vi "asc转换.vi"(11 "输入数据":u16) -> (0 "数值位 5":u8 format="%x", 1 "数值位 4":u8 format="%x", 2 "数值位 3":u8 format="%x", 3 "数值位 2":u8 format="%x")   [LabVIEW 2016]
panel:
  in  "数值 1":u8 format="%x"
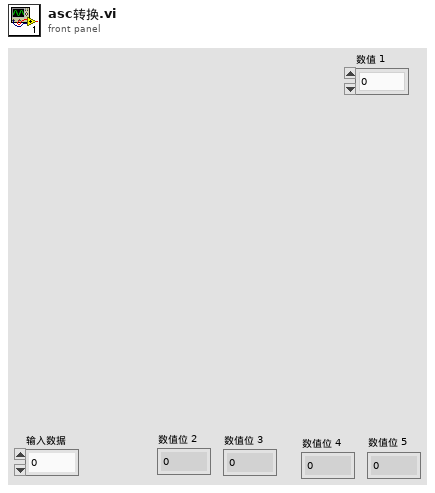
[diagram p1: front panel]
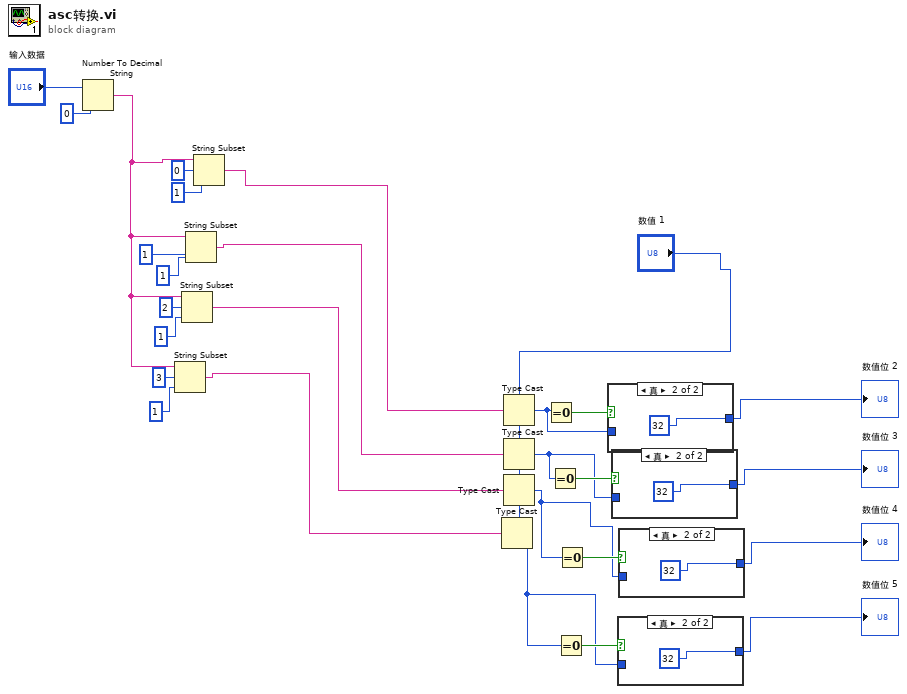
[diagram p0: block diagram]
diagram:
  n1 = Number To Decimal String(number="输入数据", width (-)=i16 0 ("宽度(-)")) -> (decimal integer string=w20:string)
  n2 = String Subset(string=w20, offset (0)=3 ("偏移量(0)"), length (rest)=1 ("长度（剩余）")) -> (substring=w14:string)
  n3 = String Subset(string=w20, offset (0)=2 ("偏移量(0)"), length (rest)=1 ("长度（剩余）")) -> (substring=w15:string)
  n4 = String Subset(string=w20, offset (0)=1 ("偏移量(0)"), length (rest)=1 ("长度（剩余）")) -> (substring=w16:string)
  n5 = String Subset(string=w20, offset (0)=0 ("偏移量(0)"), length (rest)=1 ("长度（剩余）")) -> (substring=w24:string)
  n6 = Type Cast(type="数值 1", x=w14) -> (*(type *) &x=w5:u8)
  n7 = Type Cast(type="数值 1", x=w24) -> (*(type *) &x=w11:u8)
  n8 = Type Cast(type="数值 1", x=w16) -> (*(type *) &x=w7:u8)
  n9 = Type Cast(type="数值 1", x=w15) -> (*(type *) &x=w6:u8)
  n10 = Equal To 0?(x=w11) -> (x = 0?=w13:bool)
  n11 = Equal To 0?(x=w7) -> (x = 0?=w10:bool)
  n12 = Equal To 0?(x=w5) -> (x = 0?=w8:bool)
  n13 = Equal To 0?(x=w6) -> (x = 0?=w9:bool)
  n14 = case shown="真" w13 {
    tunnel: [w29 32] -> w12
    tunnel: w11 -> [w29 _]
    frame False {
    }
    frame True {
    }
  }
  "数值位 2" <- w12
  n15 = case shown="真" w10 {
    tunnel: [w31 32] -> w4
    tunnel: w7 -> [w31 _]
    frame False {
    }
    frame True {
    }
  }
  "数值位 3" <- w4
  n16 = case shown="真" w8 {
    tunnel: [w33 32] -> w2
    tunnel: w5 -> [w33 _]
    frame False {
    }
    frame True {
    }
  }
  "数值位 5" <- w2
  n17 = case shown="真" w9 {
    tunnel: [w35 32] -> w3
    tunnel: w6 -> [w35 _]
    frame False {
    }
    frame True {
    }
  }
  "数值位 4" <- w3
